vi "Sound Player.vi"(8 "Error in":errorcluster caption="Error in (no error)", 11 "path":path caption="chemin") -> (0 "Error out":errorcluster)   [LabVIEW 2020]
doc: "Ce VI montre comment relire un fichier son directement sur les hauts-parleurs. Il utilise le VI Jouer un fichier son qui ouvre un fichier et commence à jouer les données immédiatement et de manière asynchrone (contrairement à la méthode illustrée dans l'exemple Sound File to Sound Output.vi)."
panel:
  out "Lecture en cours ?":bool
  # "Présentation :  Montre comment utiliser les fonctions de son pour lire un fichier son.\nInstructions :\n1. Spécifiez l'ID du périphérique.\n2. Exécutez le VI. Cela peut prendre plusieurs secondes pour charger le fichier et démarrer la lecture."
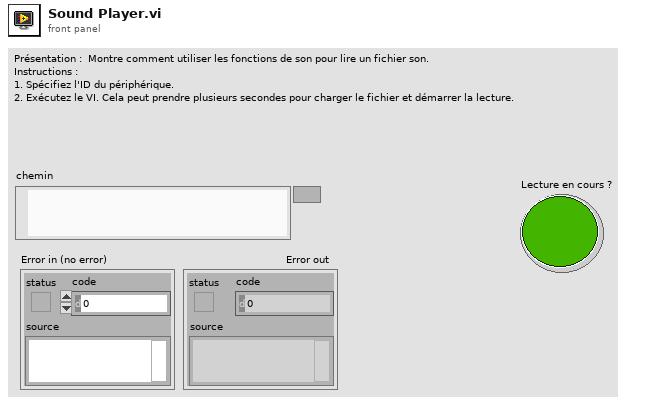
[diagram p1: front panel]
types:
  T1 = typedef "Sound Output Task ID.ctl" = u32
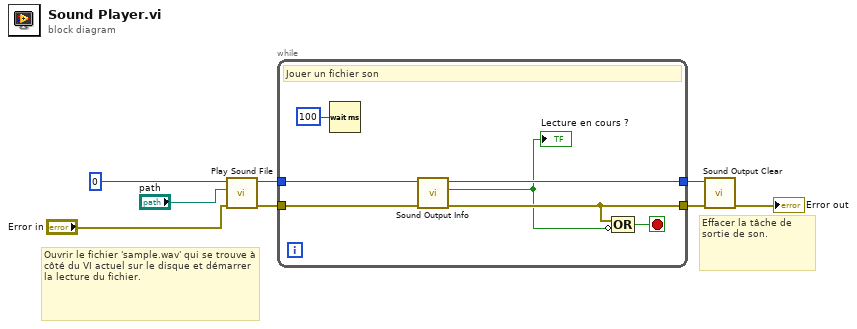
[diagram p0: block diagram]
diagram:
  # "Effacer la tâche de sortie de son."
  # "Ouvrir le fichier 'sample.wav' qui se trouve à côté du VI actuel sur le disque et démarrer la lecture du fichier."
  n1 = call <vilib>:"Play Sound File.vi"("error in (no error)"="Error in", "path"="path", "device ID"=u32 0 ("ID du périphérique")) -> ("error out"=w7:errorcluster, "task ID"=w8:T1)  [unwired: 7 in]
  n2 = while {
    tunnel: w8 -> [w10]
    tunnel: [w14] -> w5
    tunnel: w7 -> [w11]
    tunnel: [w13] -> w6
    stop <- w15 stop-if-true
    # "Jouer un fichier son"
    n3 = Wait (ms)(milliseconds to wait=u32 100) -> ()  [unwired: 1 out]
    n4 = call <vilib>:"Sound Output Info.vi"("error in (no error)"=w11, "task ID"=w10) -> ("error out"=w13:errorcluster, "is playing?"=w12:bool, "task ID out"=w14:T1)  [unwired: 6 in, 1 out]
    "Lecture en cours ?" <- w12
    n5 = Compound Arithmetic op=OR(w13, invert w12) -> (w15:bool)
  }
  n6 = call <vilib>:"Sound Output Clear.vi"("error in (no error)"=w6, "task ID"=w5) -> ("error out"=→"Error out":errorcluster)  [unwired: 9 in]
